vi "AVS_GetHandleFromSerial.vi"(0 "a_pSerial":i8) -> (4 "Output Value":i32)   [LabVIEW 2016]
uses:
  libavs.so
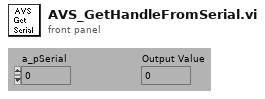
[diagram p1: front panel]
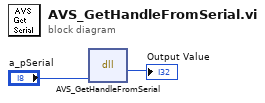
[diagram p0: block diagram]
diagram:
  n1 = dll-call lib="home/harini/tcs/ts_sedspectrometer/ss_sedspectrometer/VIs/libavs.so" fn="AVS_GetHandleFromSerial"("a_pSerial"="a_pSerial") -> ("return type"=→"Output Value":i32)  [unwired: 4 in, 2 out]
